vi "写入下次流水号.vi"(2 "error in":errorcluster, 3 "流水号":string) -> (0 "error out":errorcluster, 1 "+1流水号":string)   [LabVIEW 2016]
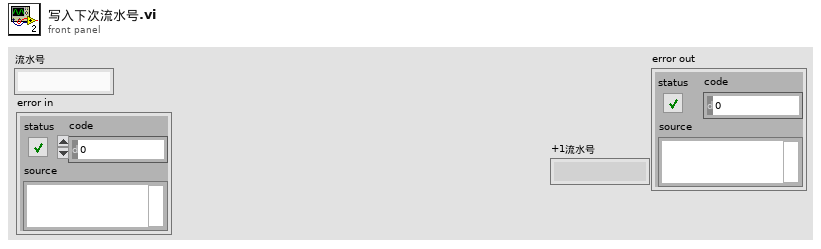
[diagram p1: front panel]
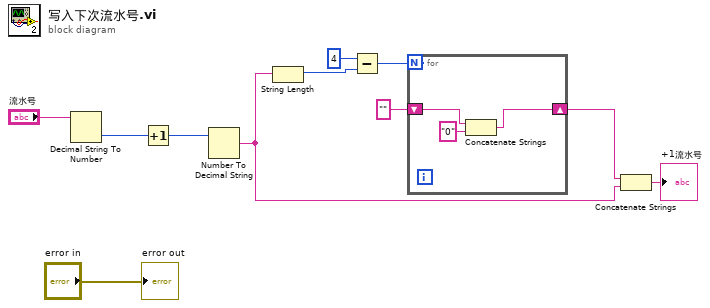
[diagram p0: block diagram]
diagram:
  n1 = Decimal String To Number(string="流水号") -> (number=w11:i32)  [unwired: 2 in, 1 out]
  n2 = Increment(x=w11) -> (x+1=w10:i32)
  n3 = Number To Decimal String(number=w10) -> (decimal integer string=w5:string)  [unwired: 1 in]
  n4 = String Length(string=w5) -> (length=w9:i32)
  n5 = Subtract(x=4, y=w9) -> (x-y=w7:i32)
  n6 = for {
    N: w7 -> [_]
    shift-right: [w13] -> w6
    shift-left: "" -> [w14]
    n7 = Concatenate Strings(w14, "0" ("string")) -> (w13:string)
  }
  n8 = Concatenate Strings(w6, w5) -> (→"+1流水号":string)
  "error out" <- "error in"
